vi "14-2.vi"() -> (3 "Resting Sand":i32)   [LabVIEW 2022 SP3, in "AoC22.lvlib"]
uses:
  AoC22.lvlib
  I32Vec2.ctl
  Regolith Cell.ctl
panel:
  in  "Vis?":bool
  in  "Speed":u32(slide)
  out "Vis":u8[][](graph)
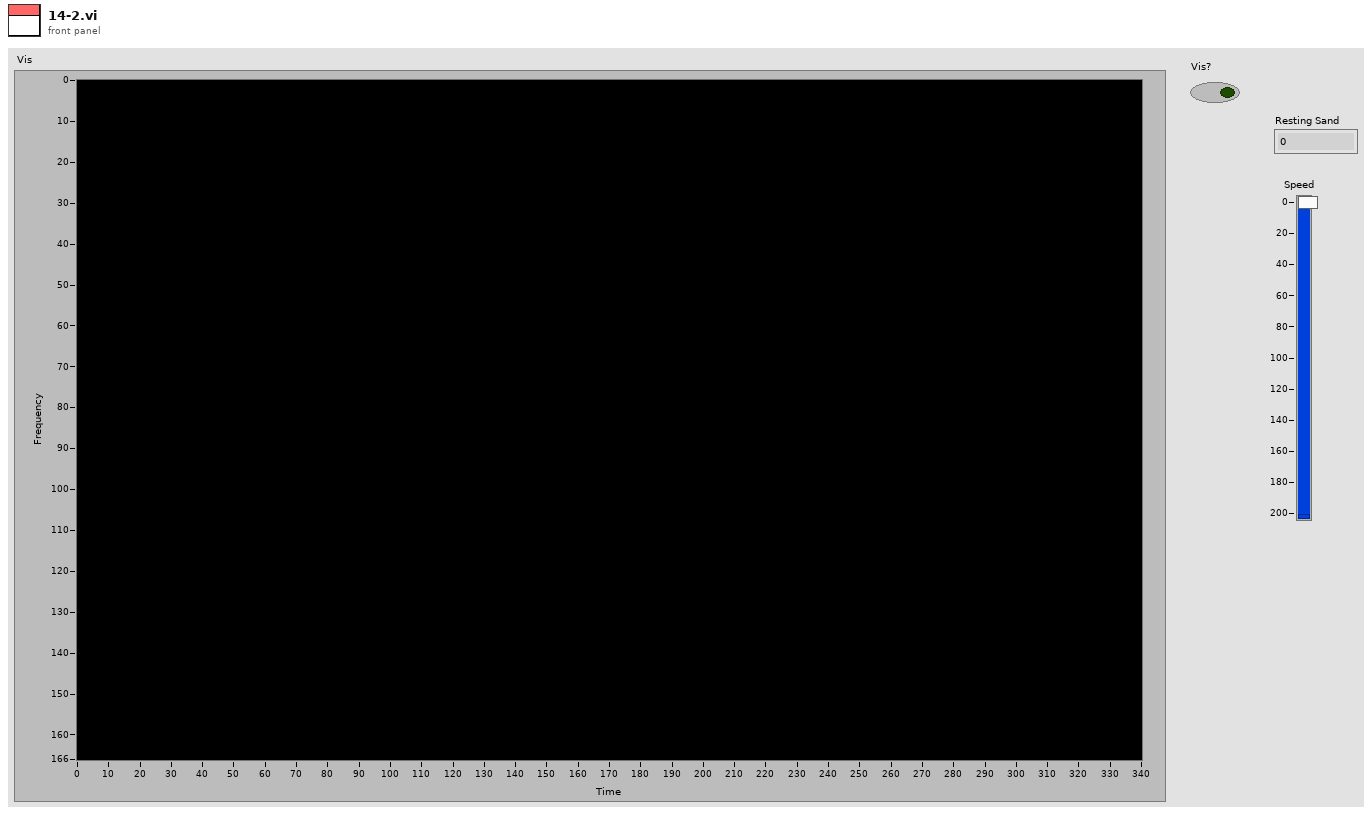
[diagram p1: front panel]
types:
  T1 = typedef "AoC22.lvlib/I32Vec2.ctl" = cluster{"X":i32, "Y":i32}
  T2 = typedef "AoC22.lvlib/Regolith Cell.ctl" = enum16{".", "#", "°", "o", "+"}
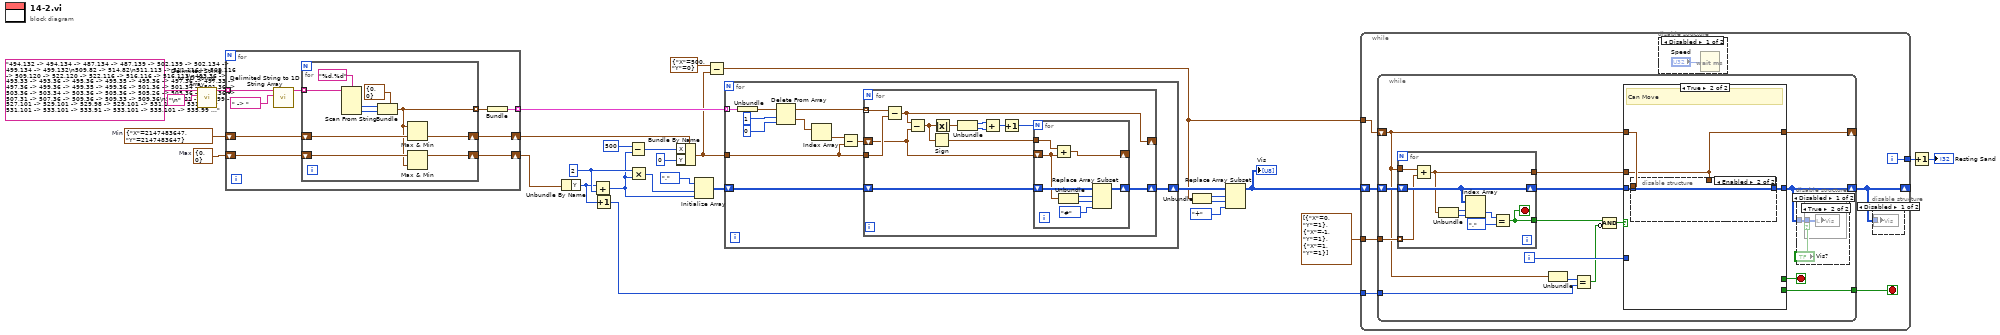
[diagram p0: block diagram]
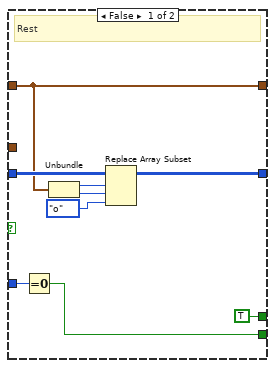
[diagram p6: hidden frame]
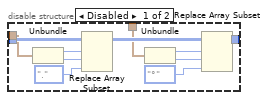
[diagram p7: hidden frame]
diagram:
  w9 = 2 ("y")
  w25 = T1 {"X"=0, "Y"=0}  # Max
  w26 = T1 {"X"=2147483647, "Y"=2147483647}  # Min
  n1 = call <vilib>:"Delimited String to 1D String Array.vi"("delimiter"="\n", "delimited string"="494,132 -> 494,134 -> 487,134 -> 487,139 -> 502,139 -> 502,134 -> 499,134 -> 499,132\n509,82 -> 514,82\n511,113 -> 511,116 -> 509,116 -> 509,120 -> 522,120 -> 522,116 -> 516,116 -> 516,113\n493,36 -> 493,33 -> 493,36 -> 495,36 -> 495,35 -> 495,36 -> 497,36 -> 497,33 -> 497,36 -> 499,36 -> 499,35 -> 499,36 -> 501,36 -> 501,34 -> 501,36 -> 503,36 -> 503,34 -> 503,36 -> 505,36 -> 505,26 -> 505,36 -> 507,36 -> 507,31 -> 507,36 -> 509,36 -> 509,33 -> 509,36\n527,101 -> 527,99 -> 527,101 -> 529,101 -> 529,98 -> 529,101 -> 531,101 -> 531,92 -> 531,101 -> 533,101 -> 533,91 -> 533,101 -> 535,101 -> 535,99 -> 535,101 -> 537,101 -> 537,100 -> 537,101 -> 539,101 -> 539,93 -> 539,101\n493,36 -> 493,33 -> 493,36 -> 495,36 -> 495,35 -> 495,36 -> 497,36 -> 497,33 -> 497,36 -> 499,36 -> 499,35 -> 499,36 -> 501,36 -> 501,34 -> 501,36 -> 503,36 -> 503,34 -> 503,36 -> 505,36 -> 505,26 -> 505,36 -> 507,36 -> 507,31 -> 507,36 -> 509,36 -> 509,33 -> 509,36\n510,65 -> 510,57 -> 510,65 -> 512,65 -> 512,63 -> 512,65 -> 514,65 -> 514,64 -> 514,65\n490,39 -> 490,42 -> 483,42 -> 483,49 -> 503,49 -> 503,42 -> 495,42 -> 495,39\n527,101 -> 527,99 -> 527,101 -> 529,101 -> 529,98 -> 529,101 -> 531,101 -> 531,92 -> 531,101 -> 533,101 -> 533,91 -> 533,101 -> 535,101 -> 535,99 -> 535,101 -> 537,101 -> 537,100 -> 537,101 -> 539,101 -> 539,93 -> 539,101\n526,150 -> 530,150\n493,36 -> 493,33 -> 493,36 -> 495,36 -> 495,35 -> 495,36 -> 497,36 -> 497,33 -> 497,36 -> 499,36 -> 499,35 -> 499,36 -> 501,36 -> 501,34 -> 501,36 -> 503,36 -> 503,34 -> 503,36 -> 505,36 -> 505,26 -> 505,36 -> 507,36 -> 507,31 -> 507,36 -> 509,36 -> 509,33 -> 509,36\n512,127 -> 516,127\n494,132 -> 494,134 -> 487,134 -> 487,139 -> 502,139 -> 502,134 -> 499,134 -> 499,132\n493,36 -> 493,33 -> 493,36 -> 495,36 -> 495,35 -> 495,36 -> 497,36 -> 497,33 -> 497,36 -> 499,36 -> 499,35 -> 499,36 -> 501,36 -> 501,34 -> 501,36 -> 503,36 -> 503,34 -> 503,36 -> 505,36 -> 505,26 -> 505,36 -> 507,36 -> 507,31 -> 507,36 -> 509,36 -> 509,33 -> 509,36\n522,153 -> 522,156 -> 515,156 -> 515,164 -> 533,164 -> 533,156 -> 528,156 -> 528,153\n493,36 -> 493,33 -> 493,36 -> 495,36 -> 495,35 -> 495,36 -> 497,36 -> 497,33 -> 497,36 -> 499,36 -> 499,35 -> 499,36 -> 501,36 -> 501,34 -> 501,36 -> 503,36 -> 503,34 -> 503,36 -> 505,36 -> 505,26 -> 505,36 -> 507,36 -> 507,31 -> 507,36 -> 509,36 -> 509,33 -> 509,36\n517,77 -> 524,77 -> 524,76\n522,153 -> 522,156 -> 515,156 -> 515,164 -> 533,164 -> 533,156 -> 528,156 -> 528,153\n493,36 -> 493,33 -> 493,36 -> 495,36 -> 495,35 -> 495,36 -> 497,36 -> 497,33 -> 497,36 -> 499,36 -> 499,35 -> 499,36 -> 501,36 -> 501,34 -> 501,36 -> 503,36 -> 503,34 -> 503,36 -> 505,36 -> 505,26 -> 505,36 -> 507,36 -> 507,31 -> 507,36 -> 509,36 -> 509,33 -> 509,36\n527,101 -> 527,99 -> 527,101 -> 529,101 -> 529,98 -> 529,101 -> 531,101 -> 531,92 -> 531,101 -> 533,101 -> 533,91 -> 533,101 -> 535,101 -> 535,99 -> 535,101 -> 537,101 -> 537,100 -> 537,101 -> 539,101 -> 539,93 -> 539,101\n529,148 -> 533,148\n521,110 -> 525,110\n493,36 -> 493,33 -> 493,36 -> 495,36 -> 495,35 -> 495,36 -> 497,36 -> 497,33 -> 497,36 -> 499,36 -> 499,35 -> 499,36 -> 501,36 -> 501,34 -> 501,36 -> 503,36 -> 503,34 -> 503,36 -> 505,36 -> 505,26 -> 505,36 -> 507,36 -> 507,31 -> 507,36 -> 509,36 -> 509,33 -> 509,36\n511,113 -> 511,116 -> 509,116 -> 509,120 -> 522,120 -> 522,116 -> 516,116 -> 516,113\n493,36 -> 493,33 -> 493,36 -> 495,36 -> 495,35 -> 495,36 -> 497,36 -> 497,33 -> 497,36 -> 499,36 -> 499,35 -> 499,36 -> 501,36 -> 501,34 -> 501,36 -> 503,36 -> 503,34 -> 503,36 -> 505,36 -> 505,26 -> 505,36 -> 507,36 -> 507,31 -> 507,36 -> 509,36 -> 509,33 -> 509,36\n493,36 -> 493,33 -> 493,36 -> 495,36 -> 495,35 -> 495,36 -> 497,36 -> 497,33 -> 497,36 -> 499,36 -> 499,35 -> 499,36 -> 501,36 -> 501,34 -> 501,36 -> 503,36 -> 503,34 -> 503,36 -> 505,36 -> 505,26 -> 505,36 -> 507,36 -> 507,31 -> 507,36 -> 509,36 -> 509,33 -> 509,36\n506,123 -> 510,123\n490,39 -> 490,42 -> 483,42 -> 483,49 -> 503,49 -> 503,42 -> 495,42 -> 495,39\n494,132 -> 494,134 -> 487,134 -> 487,139 -> 502,139 -> 502,134 -> 499,134 -> 499,132\n522,153 -> 522,156 -> 515,156 -> 515,164 -> 533,164 -> 533,156 -> 528,156 -> 528,153\n522,153 -> 522,156 -> 515,156 -> 515,164 -> 533,164 -> 533,156 -> 528,156 -> 528,153\n527,101 -> 527,99 -> 527,101 -> 529,101 -> 529,98 -> 529,101 -> 531,101 -> 531,92 -> 531,101 -> 533,101 -> 533,91 -> 533,101 -> 535,101 -> 535,99 -> 535,101 -> 537,101 -> 537,100 -> 537,101 -> 539,101 -> 539,93 -> 539,101\n510,65 -> 510,57 -> 510,65 -> 512,65 -> 512,63 -> 512,65 -> 514,65 -> 514,64 -> 514,65\n517,77 -> 524,77 -> 524,76\n520,84 -> 525,84\n506,127 -> 510,127\n522,153 -> 522,156 -> 515,156 -> 515,164 -> 533,164 -> 533,156 -> 528,156 -> 528,153\n494,132 -> 494,134 -> 487,134 -> 487,139 -> 502,139 -> 502,134 -> 499,134 -> 499,132\n494,132 -> 494,134 -> 487,134 -> 487,139 -> 502,139 -> 502,134 -> 499,134 -> 499,132\n497,23 -> 497,14 -> 497,23 -> 499,23 -> 499,16 -> 499,23 -> 501,23 -> 501,17 -> 501,23\n528,88 -> 533,88\n527,101 -> 527,99 -> 527,101 -> 529,101 -> 529,98 -> 529,101 -> 531,101 -> 531,92 -> 531,101 -> 533,101 -> 533,91 -> 533,101 -> 535,101 -> 535,99 -> 535,101 -> 537,101 -> 537,100 -> 537,101 -> 539,101 -> 539,93 -> 539,101\n497,23 -> 497,14 -> 497,23 -> 499,23 -> 499,16 -> 499,23 -> 501,23 -> 501,17 -> 501,23\n493,36 -> 493,33 -> 493,36 -> 495,36 -> 495,35 -> 495,36 -> 497,36 -> 497,33 -> 497,36 -> 499,36 -> 499,35 -> 499,36 -> 501,36 -> 501,34 -> 501,36 -> 503,36 -> 503,34 -> 503,36 -> 505,36 -> 505,26 -> 505,36 -> 507,36 -> 507,31 -> 507,36 -> 509,36 -> 509,33 -> 509,36\n527,101 -> 527,99 -> 527,101 -> 529,101 -> 529,98 -> 529,101 -> 531,101 -> 531,92 -> 531,101 -> 533,101 -> 533,91 -> 533,101 -> 535,101 -> 535,99 -> 535,101 -> 537,101 -> 537,100 -> 537,101 -> 539,101 -> 539,93 -> 539,101\n490,39 -> 490,42 -> 483,42 -> 483,49 -> 503,49 -> 503,42 -> 495,42 -> 495,39\n550,150 -> 554,150\n527,101 -> 527,99 -> 527,101 -> 529,101 -> 529,98 -> 529,101 -> 531,101 -> 531,92 -> 531,101 -> 533,101 -> 533,91 -> 533,101 -> 535,101 -> 535,99 -> 535,101 -> 537,101 -> 537,100 -> 537,101 -> 539,101 -> 539,93 -> 539,101\n493,36 -> 493,33 -> 493,36 -> 495,36 -> 495,35 -> 495,36 -> 497,36 -> 497,33 -> 497,36 -> 499,36 -> 499,35 -> 499,36 -> 501,36 -> 501,34 -> 501,36 -> 503,36 -> 503,34 -> 503,36 -> 505,36 -> 505,26 -> 505,36 -> 507,36 -> 507,31 -> 507,36 -> 509,36 -> 509,33 -> 509,36\n514,88 -> 519,88\n493,36 -> 493,33 -> 493,36 -> 495,36 -> 495,35 -> 495,36 -> 497,36 -> 497,33 -> 497,36 -> 499,36 -> 499,35 -> 499,36 -> 501,36 -> 501,34 -> 501,36 -> 503,36 -> 503,34 -> 503,36 -> 505,36 -> 505,26 -> 505,36 -> 507,36 -> 507,31 -> 507,36 -> 509,36 -> 509,33 -> 509,36\n506,84 -> 511,84\n506,52 -> 512,52 -> 512,51\n516,74 -> 520,74\n524,104 -> 528,104\n506,52 -> 512,52 -> 512,51\n511,113 -> 511,116 -> 509,116 -> 509,120 -> 522,120 -> 522,116 -> 516,116 -> 516,113\n527,106 -> 531,106\n497,23 -> 497,14 -> 497,23 -> 499,23 -> 499,16 -> 499,23 -> 501,23 -> 501,17 -> 501,23\n507,67 -> 507,68 -> 518,68 -> 518,67\n493,36 -> 493,33 -> 493,36 -> 495,36 -> 495,35 -> 495,36 -> 497,36 -> 497,33 -> 497,36 -> 499,36 -> 499,35 -> 499,36 -> 501,36 -> 501,34 -> 501,36 -> 503,36 -> 503,34 -> 503,36 -> 505,36 -> 505,26 -> 505,36 -> 507,36 -> 507,31 -> 507,36 -> 509,36 -> 509,33 -> 509,36\n538,146 -> 542,146\n497,23 -> 497,14 -> 497,23 -> 499,23 -> 499,16 -> 499,23 -> 501,23 -> 501,17 -> 501,23\n515,110 -> 519,110\n527,101 -> 527,99 -> 527,101 -> 529,101 -> 529,98 -> 529,101 -> 531,101 -> 531,92 -> 531,101 -> 533,101 -> 533,91 -> 533,101 -> 535,101 -> 535,99 -> 535,101 -> 537,101 -> 537,100 -> 537,101 -> 539,101 -> 539,93 -> 539,101\n530,108 -> 534,108\n497,23 -> 497,14 -> 497,23 -> 499,23 -> 499,16 -> 499,23 -> 501,23 -> 501,17 -> 501,23\n503,129 -> 507,129\n535,144 -> 539,144\n493,36 -> 493,33 -> 493,36 -> 495,36 -> 495,35 -> 495,36 -> 497,36 -> 497,33 -> 497,36 -> 499,36 -> 499,35 -> 499,36 -> 501,36 -> 501,34 -> 501,36 -> 503,36 -> 503,34 -> 503,36 -> 505,36 -> 505,26 -> 505,36 -> 507,36 -> 507,31 -> 507,36 -> 509,36 -> 509,33 -> 509,36\n493,36 -> 493,33 -> 493,36 -> 495,36 -> 495,35 -> 495,36 -> 497,36 -> 497,33 -> 497,36 -> 499,36 -> 499,35 -> 499,36 -> 501,36 -> 501,34 -> 501,36 -> 503,36 -> 503,34 -> 503,36 -> 505,36 -> 505,26 -> 505,36 -> 507,36 -> 507,31 -> 507,36 -> 509,36 -> 509,33 -> 509,36\n507,67 -> 507,68 -> 518,68 -> 518,67\n500,88 -> 505,88\n507,67 -> 507,68 -> 518,68 -> 518,67\n500,127 -> 504,127\n511,113 -> 511,116 -> 509,116 -> 509,120 -> 522,120 -> 522,116 -> 516,116 -> 516,113\n517,86 -> 522,86\n493,36 -> 493,33 -> 493,36 -> 495,36 -> 495,35 -> 495,36 -> 497,36 -> 497,33 -> 497,36 -> 499,36 -> 499,35 -> 499,36 -> 501,36 -> 501,34 -> 501,36 -> 503,36 -> 503,34 -> 503,36 -> 505,36 -> 505,26 -> 505,36 -> 507,36 -> 507,31 -> 507,36 -> 509,36 -> 509,33 -> 509,36\n497,23 -> 497,14 -> 497,23 -> 499,23 -> 499,16 -> 499,23 -> 501,23 -> 501,17 -> 501,23\n527,110 -> 531,110\n527,101 -> 527,99 -> 527,101 -> 529,101 -> 529,98 -> 529,101 -> 531,101 -> 531,92 -> 531,101 -> 533,101 -> 533,91 -> 533,101 -> 535,101 -> 535,99 -> 535,101 -> 537,101 -> 537,100 -> 537,101 -> 539,101 -> 539,93 -> 539,101\n513,84 -> 518,84\n510,65 -> 510,57 -> 510,65 -> 512,65 -> 512,63 -> 512,65 -> 514,65 -> 514,64 -> 514,65\n533,110 -> 537,110\n503,125 -> 507,125\n535,148 -> 539,148\n507,88 -> 512,88\n493,36 -> 493,33 -> 493,36 -> 495,36 -> 495,35 -> 495,36 -> 497,36 -> 497,33 -> 497,36 -> 499,36 -> 499,35 -> 499,36 -> 501,36 -> 501,34 -> 501,36 -> 503,36 -> 503,34 -> 503,36 -> 505,36 -> 505,26 -> 505,36 -> 507,36 -> 507,31 -> 507,36 -> 509,36 -> 509,33 -> 509,36\n527,101 -> 527,99 -> 527,101 -> 529,101 -> 529,98 -> 529,101 -> 531,101 -> 531,92 -> 531,101 -> 533,101 -> 533,91 -> 533,101 -> 535,101 -> 535,99 -> 535,101 -> 537,101 -> 537,100 -> 537,101 -> 539,101 -> 539,93 -> 539,101\n510,65 -> 510,57 -> 510,65 -> 512,65 -> 512,63 -> 512,65 -> 514,65 -> 514,64 -> 514,65\n524,108 -> 528,108\n490,39 -> 490,42 -> 483,42 -> 483,49 -> 503,49 -> 503,42 -> 495,42 -> 495,39\n527,101 -> 527,99 -> 527,101 -> 529,101 -> 529,98 -> 529,101 -> 531,101 -> 531,92 -> 531,101 -> 533,101 -> 533,91 -> 533,101 -> 535,101 -> 535,99 -> 535,101 -> 537,101 -> 537,100 -> 537,101 -> 539,101 -> 539,93 -> 539,101\n544,150 -> 548,150\n524,86 -> 529,86\n512,80 -> 517,80\n527,101 -> 527,99 -> 527,101 -> 529,101 -> 529,98 -> 529,101 -> 531,101 -> 531,92 -> 531,101 -> 533,101 -> 533,91 -> 533,101 -> 535,101 -> 535,99 -> 535,101 -> 537,101 -> 537,100 -> 537,101 -> 539,101 -> 539,93 -> 539,101\n490,39 -> 490,42 -> 483,42 -> 483,49 -> 503,49 -> 503,42 -> 495,42 -> 495,39\n521,106 -> 525,106\n522,153 -> 522,156 -> 515,156 -> 515,164 -> 533,164 -> 533,156 -> 528,156 -> 528,153\n493,36 -> 493,33 -> 493,36 -> 495,36 -> 495,35 -> 495,36 -> 497,36 -> 497,33 -> 497,36 -> 499,36 -> 499,35 -> 499,36 -> 501,36 -> 501,34 -> 501,36 -> 503,36 -> 503,34 -> 503,36 -> 505,36 -> 505,26 -> 505,36 -> 507,36 -> 507,31 -> 507,36 -> 509,36 -> 509,33 -> 509,36\n527,101 -> 527,99 -> 527,101 -> 529,101 -> 529,98 -> 529,101 -> 531,101 -> 531,92 -> 531,101 -> 533,101 -> 533,91 -> 533,101 -> 535,101 -> 535,99 -> 535,101 -> 537,101 -> 537,100 -> 537,101 -> 539,101 -> 539,93 -> 539,101\n503,86 -> 508,86\n497,23 -> 497,14 -> 497,23 -> 499,23 -> 499,16 -> 499,23 -> 501,23 -> 501,17 -> 501,23\n509,125 -> 513,125\n527,101 -> 527,99 -> 527,101 -> 529,101 -> 529,98 -> 529,101 -> 531,101 -> 531,92 -> 531,101 -> 533,101 -> 533,91 -> 533,101 -> 535,101 -> 535,99 -> 535,101 -> 537,101 -> 537,100 -> 537,101 -> 539,101 -> 539,93 -> 539,101\n532,146 -> 536,146\n516,82 -> 521,82\n510,65 -> 510,57 -> 510,65 -> 512,65 -> 512,63 -> 512,65 -> 514,65 -> 514,64 -> 514,65\n493,36 -> 493,33 -> 493,36 -> 495,36 -> 495,35 -> 495,36 -> 497,36 -> 497,33 -> 497,36 -> 499,36 -> 499,35 -> 499,36 -> 501,36 -> 501,34 -> 501,36 -> 503,36 -> 503,34 -> 503,36 -> 505,36 -> 505,26 -> 505,36 -> 507,36 -> 507,31 -> 507,36 -> 509,36 -> 509,33 -> 509,36\n509,129 -> 513,129\n541,148 -> 545,148\n490,39 -> 490,42 -> 483,42 -> 483,49 -> 503,49 -> 503,42 -> 495,42 -> 495,39\n494,132 -> 494,134 -> 487,134 -> 487,139 -> 502,139 -> 502,134 -> 499,134 -> 499,132\n497,23 -> 497,14 -> 497,23 -> 499,23 -> 499,16 -> 499,23 -> 501,23 -> 501,17 -> 501,23\n493,36 -> 493,33 -> 493,36 -> 495,36 -> 495,35 -> 495,36 -> 497,36 -> 497,33 -> 497,36 -> 499,36 -> 499,35 -> 499,36 -> 501,36 -> 501,34 -> 501,36 -> 503,36 -> 503,34 -> 503,36 -> 505,36 -> 505,26 -> 505,36 -> 507,36 -> 507,31 -> 507,36 -> 509,36 -> 509,33 -> 509,36\n511,113 -> 511,116 -> 509,116 -> 509,120 -> 522,120 -> 522,116 -> 516,116 -> 516,113\n490,39 -> 490,42 -> 483,42 -> 483,49 -> 503,49 -> 503,42 -> 495,42 -> 495,39\n541,144 -> 545,144\n493,36 -> 493,33 -> 493,36 -> 495,36 -> 495,35 -> 495,36 -> 497,36 -> 497,33 -> 497,36 -> 499,36 -> 499,35 -> 499,36 -> 501,36 -> 501,34 -> 501,36 -> 503,36 -> 503,34 -> 503,36 -> 505,36 -> 505,26 -> 505,36 -> 507,36 -> 507,31 -> 507,36 -> 509,36 -> 509,33 -> 509,36\n493,36 -> 493,33 -> 493,36 -> 495,36 -> 495,35 -> 495,36 -> 497,36 -> 497,33 -> 497,36 -> 499,36 -> 499,35 -> 499,36 -> 501,36 -> 501,34 -> 501,36 -> 503,36 -> 503,34 -> 503,36 -> 505,36 -> 505,26 -> 505,36 -> 507,36 -> 507,31 -> 507,36 -> 509,36 -> 509,33 -> 509,36\n511,113 -> 511,116 -> 509,116 -> 509,120 -> 522,120 -> 522,116 -> 516,116 -> 516,113\n538,150 -> 542,150\n510,65 -> 510,57 -> 510,65 -> 512,65 -> 512,63 -> 512,65 -> 514,65 -> 514,64 -> 514,65\n511,113 -> 511,116 -> 509,116 -> 509,120 -> 522,120 -> 522,116 -> 516,116 -> 516,113\n527,101 -> 527,99 -> 527,101 -> 529,101 -> 529,98 -> 529,101 -> 531,101 -> 531,92 -> 531,101 -> 533,101 -> 533,91 -> 533,101 -> 535,101 -> 535,99 -> 535,101 -> 537,101 -> 537,100 -> 537,101 -> 539,101 -> 539,93 -> 539,101\n515,129 -> 519,129\n493,36 -> 493,33 -> 493,36 -> 495,36 -> 495,35 -> 495,36 -> 497,36 -> 497,33 -> 497,36 -> 499,36 -> 499,35 -> 499,36 -> 501,36 -> 501,34 -> 501,36 -> 503,36 -> 503,34 -> 503,36 -> 505,36 -> 505,26 -> 505,36 -> 507,36 -> 507,31 -> 507,36 -> 509,36 -> 509,33 -> 509,36\n510,65 -> 510,57 -> 510,65 -> 512,65 -> 512,63 -> 512,65 -> 514,65 -> 514,64 -> 514,65\n522,153 -> 522,156 -> 515,156 -> 515,164 -> 533,164 -> 533,156 -> 528,156 -> 528,153\n493,36 -> 493,33 -> 493,36 -> 495,36 -> 495,35 -> 495,36 -> 497,36 -> 497,33 -> 497,36 -> 499,36 -> 499,35 -> 499,36 -> 501,36 -> 501,34 -> 501,36 -> 503,36 -> 503,34 -> 503,36 -> 505,36 -> 505,26 -> 505,36 -> 507,36 -> 507,31 -> 507,36 -> 509,36 -> 509,33 -> 509,36\n510,86 -> 515,86\n527,101 -> 527,99 -> 527,101 -> 529,101 -> 529,98 -> 529,101 -> 531,101 -> 531,92 -> 531,101 -> 533,101 -> 533,91 -> 533,101 -> 535,101 -> 535,99 -> 535,101 -> 537,101 -> 537,100 -> 537,101 -> 539,101 -> 539,93 -> 539,101\n494,132 -> 494,134 -> 487,134 -> 487,139 -> 502,139 -> 502,134 -> 499,134 -> 499,132\n521,88 -> 526,88\n527,101 -> 527,99 -> 527,101 -> 529,101 -> 529,98 -> 529,101 -> 531,101 -> 531,92 -> 531,101 -> 533,101 -> 533,91 -> 533,101 -> 535,101 -> 535,99 -> 535,101 -> 537,101 -> 537,100 -> 537,101 -> 539,101 -> 539,93 -> 539,101\n510,65 -> 510,57 -> 510,65 -> 512,65 -> 512,63 -> 512,65 -> 514,65 -> 514,64 -> 514,65\n497,129 -> 501,129\n527,101 -> 527,99 -> 527,101 -> 529,101 -> 529,98 -> 529,101 -> 531,101 -> 531,92 -> 531,101 -> 533,101 -> 533,91 -> 533,101 -> 535,101 -> 535,99 -> 535,101 -> 537,101 -> 537,100 -> 537,101 -> 539,101 -> 539,93 -> 539,101\n532,150 -> 536,150\n493,36 -> 493,33 -> 493,36 -> 495,36 -> 495,35 -> 495,36 -> 497,36 -> 497,33 -> 497,36 -> 499,36 -> 499,35 -> 499,36 -> 501,36 -> 501,34 -> 501,36 -> 503,36 -> 503,34 -> 503,36 -> 505,36 -> 505,26 -> 505,36 -> 507,36 -> 507,31 -> 507,36 -> 509,36 -> 509,33 -> 509,36\n527,101 -> 527,99 -> 527,101 -> 529,101 -> 529,98 -> 529,101 -> 531,101 -> 531,92 -> 531,101 -> 533,101 -> 533,91 -> 533,101 -> 535,101 -> 535,99 -> 535,101 -> 537,101 -> 537,100 -> 537,101 -> 539,101 -> 539,93 -> 539,101\n547,148 -> 551,148\n493,36 -> 493,33 -> 493,36 -> 495,36 -> 495,35 -> 495,36 -> 497,36 -> 497,33 -> 497,36 -> 499,36 -> 499,35 -> 499,36 -> 501,36 -> 501,34 -> 501,36 -> 503,36 -> 503,34 -> 503,36 -> 505,36 -> 505,26 -> 505,36 -> 507,36 -> 507,31 -> 507,36 -> 509,36 -> 509,33 -> 509,36\n518,108 -> 522,108\n544,146 -> 548,146\n527,101 -> 527,99 -> 527,101 -> 529,101 -> 529,98 -> 529,101 -> 531,101 -> 531,92 -> 531,101 -> 533,101 -> 533,91 -> 533,101 -> 535,101 -> 535,99 -> 535,101 -> 537,101 -> 537,100 -> 537,101 -> 539,101 -> 539,93 -> 539,101\n538,142 -> 542,142") -> ("string array"=w27:string[])  [unwired: 9 in]
  n2 = for {
    tunnel: w27 -> [w38] mode=indexing
    tunnel: [w34] -> w21 mode=indexing
    shift-right: [w31] -> w23
    shift-left: w26 -> [w32]
    shift-right: [w30] -> w24
    shift-left: w25 -> [w33]
    n3 = call <vilib>:"Delimited String to 1D String Array.vi"("delimiter"=" -> ", "delimited string"=w38) -> ("string array"=w36:string[])  [unwired: 9 in]
    n4 = for {
      tunnel: w36 -> [w48] mode=indexing
      tunnel: [w40] -> w35 mode=indexing
      shift-right: [w39] -> w30
      shift-left: w33 -> [w41]
      shift-right: [w42] -> w31
      shift-left: w32 -> [w43]
      n5 = Scan From String(format string="%d,%d", input string=w48) -> (output 1=w45:i32, output 2=w44:i32)  [unwired: 4 in, 3 out]
      n6 = Bundle(cluster=T1 {"X"=0, "Y"=0} ("I32Vec2"), "X"=w45, "Y"=w44) -> (w40:T1)
      n7 = Max & Min(x=w40, y=w43) -> (min(x,y)=w42:T1)  [unwired: 1 out]
      n8 = Max & Min(x=w41, y=w40) -> (max(x,y)=w39:T1)  [unwired: 1 out]
    }
    n9 = Bundle(w35) -> (w34:cluster{T1[]})  [unwired: 1 in]
  }
  n10 = Unbundle By Name(w24) -> ("Y"=w3:i32)
  n11 = Add(x=w3, y=w9) -> (x+y=w7:i32)
  n12 = Increment(x=w3) -> (x+1=w2:i32)
  n13 = Subtract(x=500 ("X"), y=w7) -> (x-y=w4:i32)
  n14 = Multiply(x=w9, y=w7) -> (x*y=w6:i32)
  n15 = Bundle By Name(cluster=w23, "X"=w4, "Y"=0) -> (w17:T1)
  n16 = Initialize Array(Regolith_Cell."." ("Regolith Cell"), w6, w7) -> (w19:T2[][])
  n17 = Subtract(x=T1 {"X"=500, "Y"=0} ("I32Vec2"), y=w17) -> (x-y=w10:T1)
  n18 = for {
    tunnel: w17 -> [w51]
    tunnel: w21 -> [w59] mode=indexing
    shift-right: [w56] -> w18
    shift-left: w19 -> [w57]
    n19 = Unbundle(w59) -> (w58:T1[])
    n20 = Delete From Array(array=w58, length=1, index=0) -> (deleted portion=w52:T1[], array with subset deleted=w55:T1[])
    n21 = Index Array(array=w52) -> (element=w49:T1)  [unwired: 1 in]
    n22 = Subtract(x=w49, y=w51) -> (x-y=w50:T1)
    n23 = for {
      tunnel: w55 -> [w72] mode=indexing
      tunnel: w51 -> [w62]
      shift-right: [w70] -> w56
      shift-left: w57 -> [w71]
      shift-right: [w69] -> _
      shift-left: w50 -> [w60]
      n24 = Subtract(x=w72, y=w62) -> (x-y=w69:T1)
      n25 = Subtract(x=w69, y=w60) -> (x-y=w68:T1)
      n26 = Sign(1:w68) -> (0:w61:T1)
      n27 = Absolute Value(x=w68) -> (abs(x)=w67:T1)
      n28 = Unbundle(w67) -> ("X"=w66:i32, "Y"=w65:i32)
      n29 = Add(x=w66, y=w65) -> (x+y=w64:i32)
      n30 = Increment(x=w64) -> (x+1=w63:i32)
      n31 = for {
        N: w63 -> [_]
        shift-right: [w78] -> w70
        shift-left: w71 -> [w80]
        shift-right: [w73] -> _
        shift-left: w60 -> [w75]
        tunnel: w61 -> [w74]
        n32 = Add(x=w74, y=w75) -> (x+y=w73:T1)
        n33 = Unbundle(w75) -> ("X"=w77:i32, "Y"=w76:i32)
        n34 = Replace Array Subset(array=w80, new element=Regolith_Cell."#" ("new element/subarray"), index (row)=w77, index (col)=w76) -> (w78:T2[][])
      }
    }
  }
  n35 = Unbundle(w10) -> ("X"=w16:i32, "Y"=w15:i32)
  n36 = Replace Array Subset(array=w18, new element=Regolith_Cell."+" ("new element/subarray"), index (row)=w16, index (col)=w15) -> (w13:T2[][])
  "Vis" <- w13
  n37 = while {
    shift-right: [w81] -> _
    shift-left: w13 -> [w86]
    tunnel: T1[] [{"X"=0, "Y"=1}, {"X"=-1, "Y"=1}, {"X"=1, "Y"=1}] -> [w85]
    tunnel: w2 -> [w84]
    tunnel: w10 -> [w82]
    tunnel: [w87] -> w11
    i -> [w87]
    stop <- w83 stop-if-true
    n38 = while {
      shift-right: [w98] -> w81
      shift-left: w86 -> [w104]
      tunnel: w85 -> [w103]
      tunnel: w84 -> [w93]
      shift-right: [w99] -> _
      shift-left: w82 -> [w90]
      tunnel: [w96] -> w83
      i -> [w97]
      stop <- w100 stop-if-true
      n39 = for {
        tunnel: w90 -> [w136]
        shift-right: [w139] -> w101
        shift-left: w104 -> [w139]
        tunnel: w103 -> [w135] mode=indexing
        tunnel: [w134] -> w102
        tunnel: [w133] -> w95
        stop <- w134 stop-if-true
        n40 = Add(x=w136, y=w135) -> (x+y=w133:T1)
        n41 = Unbundle(w133) -> ("X"=w141:i32, "Y"=w140:i32)
        n42 = Index Array(array=w139, index (row)=w141, index (col)=w140) -> (element=w138:T2)
        n43 = Equal?(x=w138, y=Regolith_Cell.".") -> (x = y?=w134:bool)
      }
      n44 = Unbundle(w90) -> ("Y"=w94:i32)  [unwired: 1 out]
      n45 = Equal?(x=w94, y=w93) -> (x = y?=w91:bool)
      n46 = Compound Arithmetic op=AND(w102, invert w91) -> (w92:bool)
      n47 = case shown="True" w92 {
        tunnel: w95 -> [_ w117]
        tunnel: w101 -> [w113 w120]
        tunnel: w90 -> [w110 w119]
        tunnel: [w111 w118] -> w98
        tunnel: [w108 _] -> w96
        tunnel: [TRUE _] -> w100
        tunnel: [w110 w117] -> w99
        tunnel: w97 -> [w109 _]
        frame False {
          # "Rest"
          n48 = Equal To 0?(x=w109) -> (x = 0?=w108:bool)
          n49 = Unbundle(w110) -> ("X"=w115:i32, "Y"=w114:i32)
          n50 = Replace Array Subset(array=w113, new element=Regolith_Cell."o" ("new element/subarray"), index (row)=w115, index (col)=w114) -> (w111:T2[][])
        }
        frame True {
          # "Can Move"
          n51 = disable-structure shown="Enabled" {
            disable-tunnel: w120 -> [w131 w132]
            disable-tunnel: w119 -> [w128 _]
            disable-tunnel: [w123 w132] -> w118
            disable-tunnel: w117 -> [w121 _]
            frame Disabled {
              n52 = Unbundle(w128) -> ("X"=w130:i32, "Y"=w129:i32)
              n53 = Replace Array Subset(array=w131, new element=Regolith_Cell."." ("new element/subarray"), index (row)=w130, index (col)=w129) -> (w124:T2[][])
              n54 = Unbundle(w121) -> ("X"=w125:i32, "Y"=w122:i32)
              n55 = Replace Array Subset(array=w124, new element=Regolith_Cell."°" ("new element/subarray"), index (row)=w125, index (col)=w122) -> (w123:T2[][])
            }
            frame Enabled {
            }
          }
        }
      }
      n56 = disable-structure shown="Disabled" {
        disable-tunnel: w98 -> [w106 _]
        frame Disabled {
          n57 = case shown="True" "Vis?" {
            tunnel: w106 -> [_ w107]
            frame False {
            }
            frame True {
              n58 = local write "Vis"(w107) -> ()
            }
          }
        }
        frame Enabled {
        }
      }
    }
    n59 = disable-structure shown="Disabled" {
      frame Disabled {
        n60 = Wait (ms)(milliseconds to wait="Speed") -> ()  [unwired: 1 out]
      }
      frame Enabled {
      }
    }
    n61 = disable-structure shown="Disabled" {
      disable-tunnel: w81 -> [w89 _]
      frame Disabled {
        n62 = local write "Vis"(w89) -> ()
      }
      frame Enabled {
      }
    }
  }
  n63 = Increment(x=w11) -> (x+1=→"Resting Sand":i32)
